vi "make_folder_and_filename.vi"(8 "error in (no error)":errorcluster, 10 "Storage parameters":T1, 11 "Fileno":i32) -> (0 "error out":errorcluster, 3 "Path":path)   [LabVIEW 2010]
uses:
  typedefs/storage_parameters_cluster.ctl
panel:
  # "_0000.txt"
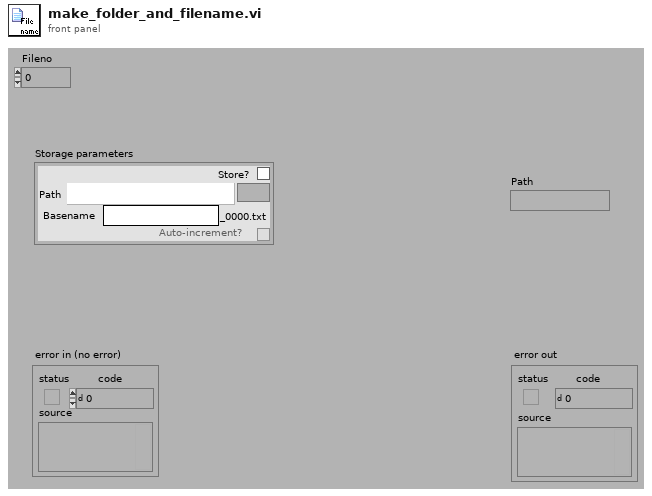
[diagram p1: front panel]
types:
  T1 = typedef "storage_parameters_cluster.ctl" = cluster{"Store?":bool, "Path":path, "Basename":string, "Auto-increment?":bool}
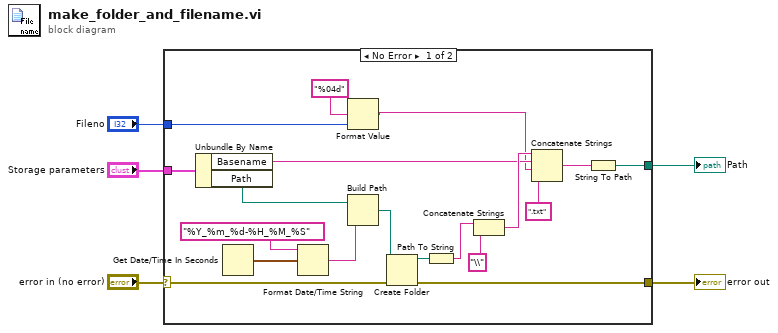
[diagram p0: block diagram]
diagram:
  n1 = case shown="No Error" "error in (no error)" {
    selector: "error in (no error)" -> [w15 w25]
    tunnel: [w14 w25] -> w4
    tunnel: "Storage parameters" -> [w22 _]
    tunnel: [w23 _] -> w2
    tunnel: "Fileno" -> [w7 _]
    frame No Error {
      n2 = Unbundle By Name(w22) -> ("Basename"=w10:string, "Path"=w19:path)
      n3 = Get Date/Time In Seconds() -> (seconds since 1Jan1904=w17:timestamp)
      n4 = Format Date/Time String(time format string (%c)="%Y_%m_%d-%H_%M_%S", seconds (now)=w17) -> (date/time string=w16:string)  [unwired: 1 in]
      n5 = Format Value(format string="%04d", value (0)=w7) -> (output string=w8:string)  [unwired: 1 in]
      n6 = Build Path(base path=w19, name or relative path=w16) -> (appended path=w13:path)
      n7 = Create Folder(path (use dialog)=w13, error in=w15) -> (created path=w12:path, error out=w14:errorcluster)  [unwired: 1 in, 1 out]
      n8 = Path To String(path=w12) -> (string=w21:string)
      n9 = Concatenate Strings(w21, "\\" ("string")) -> (w11:string)
      n10 = Concatenate Strings(w11, w10, w8, ".txt" ("string")) -> (w24:string)
      n11 = String To Path(string=w24) -> (path=w23:path)
    }
    frame Error {
    }
  }
  "error out" <- w4
  "Path" <- w2
